vi "ParseScriptArray2Steps.vi"(0 "Tree Ref in":refnum<vi>, 1 "Config Cluster out":T1, 5 "Script Array":string[](array[string]), 7 "Conditional Array out":bool[](array[boolean]), 9 "Attended? Array":bool[](array[boolean]), 11 "error in":errorcluster) -> (4 "Tree Ref out":refnum<vi>, 6 "Steps with Params":T2[](array[typedef]), 15 "error out":errorcluster)   [LabVIEW 2010]
doc: "This VI takes a \"logical\" test sequence array (script array) and collects the information related to that step so that all information is saved into a file or the Builder can use it to create the TestStand steps"
uses:
  SeqBuilder/Ctls/SeqStepTypeDef.ctl
  TestComponents.ctl
  FilePaths.ctl
  Config cluster.ctl
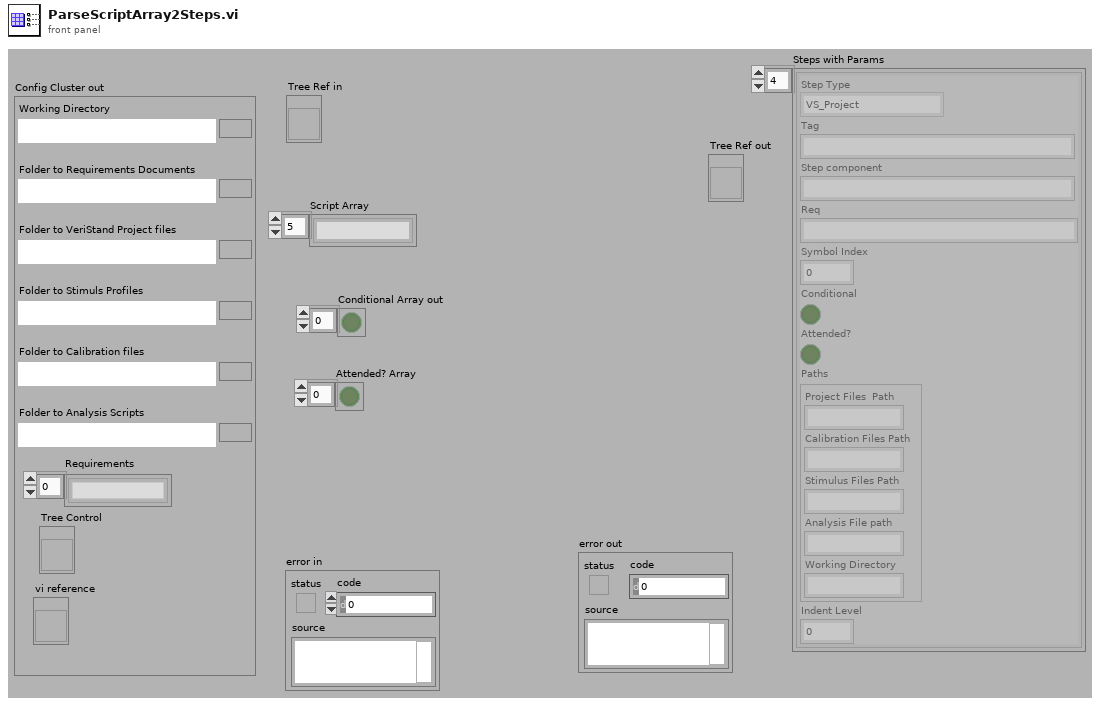
[diagram p1: front panel]
types:
  T1 = typedef "Config cluster.ctl" = cluster{"Working Directory":path, "Folder to Requirements Documents":path, "Folder to VeriStand Project files":path, "Folder to Stimuls Profiles":path, "Folder to Calibration files":path, "Folder to Analysis Scripts":path, "Requirements":string[], "Tree Control":refnum<vi>, "vi reference":refnum<vi>}
  T2 = typedef "SeqStepTypeDef.ctl" = cluster{"Step Type":T3, "Tag":string, "Step component":string, "Req":string, "Symbol Index":i32, "Conditional":bool, "Attended?":bool, "Paths":T4, "Indent Level":i32}
  T3 = typedef "TestComponents.ctl" = enum16{"Script", "Test Procedure", "VS_Project", "Calibration File", "Stimulus Profile", "Analysis Script"}
  T4 = typedef "FilePaths.ctl" = cluster{"Project Files  Path":string, "Calibration Files Path":string, "Stimulus Files Path":string, "Analysis File path":string, "Working Directory":string}
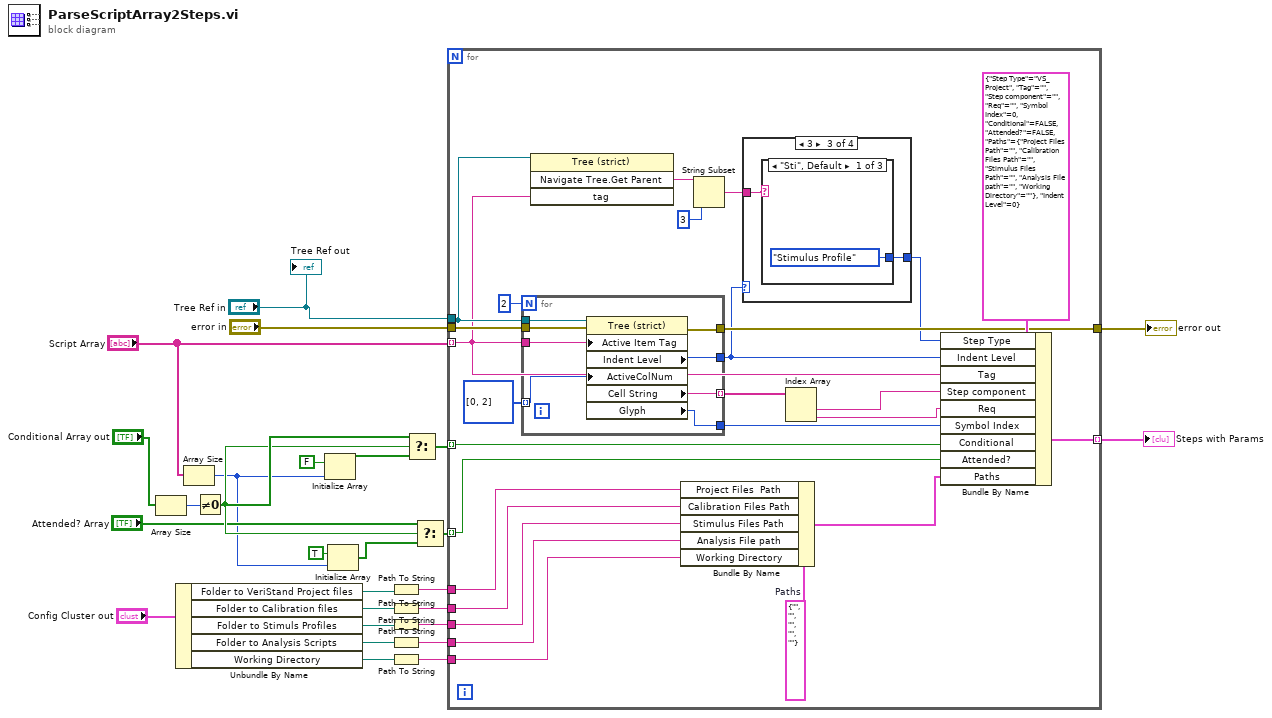
[diagram p0: block diagram]
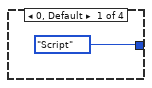
[diagram p2: hidden frame]
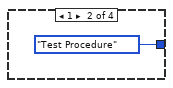
[diagram p3: hidden frame]
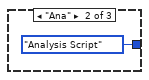
[diagram p4: hidden frame]
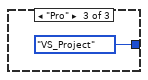
[diagram p5: hidden frame]
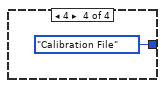
[diagram p6: hidden frame]
diagram:
  n1 = Array Size(array="Conditional Array out") -> (size(s)=w23:i32)
  n2 = Unbundle By Name("Config Cluster out") -> ("Folder to VeriStand Project files"=w10:path, "Folder to Calibration files"=w9:path, "Folder to Stimuls Profiles"=w8:path, "Folder to Analysis Scripts"=w7:path, "Working Directory"=w6:path)
  n3 = Array Size(array="Script Array") -> (size(s)=w14:i32)
  n4 = Not Equal To 0?(x=w23) -> (x != 0?=w18:bool)
  n5 = Initialize Array(FALSE ("element"), w14) -> (w16:bool[])
  n6 = Initialize Array(TRUE ("element"), w14) -> (w12:bool[])
  n7 = Path To String(path=w10) -> (string=w5:string)
  n8 = Path To String(path=w9) -> (string=w4:string)
  n9 = Path To String(path=w8) -> (string=w3:string)
  n10 = Path To String(path=w7) -> (string=w2:string)
  n11 = Path To String(path=w6) -> (string=w1:string)
  n12 = Select(t="Conditional Array out", s=w18, f=w16) -> (s? t:f=w21:bool[])
  n13 = Select(t="Attended? Array", s=w18, f=w12) -> (s? t:f=w15:bool[])
  n14 = for {
    tunnel: "Tree Ref in" -> [w42]
    tunnel: "Script Array" -> [w41] mode=indexing
    tunnel: [w52] -> w24 mode=indexing
    tunnel: "error in" -> [w47]
    tunnel: [w46] -> w25
    tunnel: w21 -> [w44] mode=indexing
    tunnel: w15 -> [w43] mode=indexing
    tunnel: w5 -> [w35]
    tunnel: w4 -> [w34]
    tunnel: w3 -> [w33]
    tunnel: w2 -> [w32]
    tunnel: w1 -> [w31]
    w37 = T4 {"Project Files  Path"="", "Calibration Files Path"="", "Stimulus Files Path"="", "Analysis File path"="", "Working Directory"=""}  # Paths
    n15 = for {
      N: 2 -> [_]
      tunnel: w42 -> [w69]
      tunnel: [w68] -> w29
      tunnel: w41 -> [w67]
      tunnel: [w66] -> w51 mode=indexing
      tunnel: w47 -> [w65]
      tunnel: [w64] -> w46
      tunnel: [w63] -> w45
      tunnel: i32[] [0, 2] -> [w62] mode=indexing
      n16 = property class="Tree (strict)"(reference=w69, error in=w65, "Active Item Tag"=w67, "ActiveColNum"=w62) -> (error out=w64:errorcluster, "Indent Level"=w68:i32, "Cell String"=w66:string, "Glyph"=w63:i32)  [unwired: 1 out]
    }
    n17 = invoke class="Tree (strict)" method="Navigate Tree.Get Parent"(reference=w42, "tag"=w41) -> ("Navigate Tree:Get Parent"=w40:string)  [unwired: 2 in, 3 out]
    n18 = Bundle By Name(cluster=w37, "Project Files  Path"=w35, "Calibration Files Path"=w34, "Stimulus Files Path"=w33, "Analysis File path"=w32, "Working Directory"=w31) -> (w36:T4)
    n19 = String Subset(string=w40, length (rest)=3 ("length (rest)")) -> (substring=w38:string)  [unwired: 1 in]
    n20 = case shown="3" w29 {
      tunnel: [TestComponents."Script" ("Step Type") TestComponents."Test Procedure" ("Step Type") w56 TestComponents."Calibration File" ("Step Type")] -> w30
      tunnel: w38 -> [_ _ w57 _]
      frame 0, Default {
      }
      frame 1 {
      }
      frame 3 {
        n21 = case shown="\"Sti\", Default" w57 {
          tunnel: [TestComponents."Stimulus Profile" ("Step Type") TestComponents."Analysis Script" ("Step Type") TestComponents."VS_Project" ("Step Type")] -> w56
          frame "Sti", Default {
          }
          frame "Ana" {
          }
          frame "Pro" {
          }
        }
      }
      frame 4 {
      }
    }
    n22 = Index Array(array=w51) -> (element #1=w50:string, element #2=w49:string)  [unwired: 2 in]
    n23 = Bundle By Name(cluster=T2 {"Step Type"=enum."VS_Project", "Tag"="", "Step component"="", "Req"="", "Symbol Index"=0, "Conditional"=FALSE, "Attended?"=FALSE, "Paths"={"Project Files  Path"="", "Calibration Files Path"="", "Stimulus Files Path"="", "Analysis File path"="", "Working Directory"=""}, "Indent Level"=0} ("Step"), "Step Type"=w30, "Indent Level"=w29, "Tag"=w41, "Step component"=w50, "Req"=w49, "Symbol Index"=w45, "Conditional"=w44, "Attended?"=w43, "Paths"=w36) -> (w52:T2)
  }
  "error out" <- w25
  "Steps with Params" <- w24
  "Tree Ref out" <- "Tree Ref in"
